vi "UTILITY Create Default File.vi"(8 "Error In":errorcluster, 10 "Default File":string[][](array[string]), 11 "Initial DOE Config":path) -> (0 "Error Out":errorcluster, 3 "new file path (Not A Path if cancelled)":path)   [LabVIEW 2018]
uses:
  <vilib>/Utility/file.llb/Write Delimited Spreadsheet (string).vi
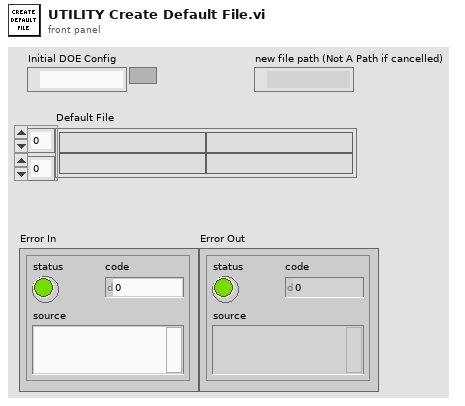
[diagram p1: front panel]
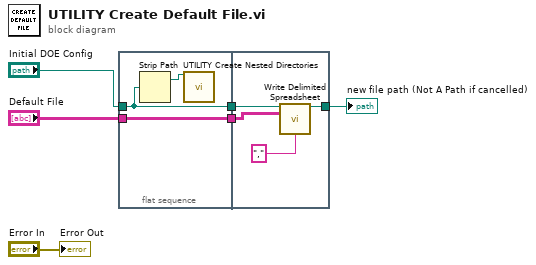
[diagram p0: block diagram]
diagram:
  n1 = flat-sequence {
    tunnel: "Initial DOE Config" -> [w8]
    tunnel: [w8] -> w3
    tunnel: "Default File" -> [w7]
    tunnel: [w7] -> w1
    tunnel: [w13] -> w6
    tunnel: w3 -> [w12]
    tunnel: w1 -> [w10]
    frame #0 {
      n2 = Strip Path(path=w8) -> (stripped path=w9:path)  [unwired: 1 out]
      n3 = call "UTILITY Create Nested Directories.vi"("path to create"=w9) -> ()  [unwired: 12 in, 3 out]
    }
    frame #1 {
      n4 = call-poly <vilib>:"Write Delimited Spreadsheet.vi"("file path (dialog if empty)"=w12, "2D data"=w10, "delimiter (\\t)"="," ("delimiter (\\t)")) -> ("new file path (Not A Path if cancelled)"=w13:path)  [unwired: 11 in, 1 out]
    }
  }
  "new file path (Not A Path if cancelled)" <- w6
  "Error Out" <- "Error In"
